vi "Cutoff Small Parts.vi"(8 "error in":errorcluster, 10 "Cutoff":dbl, 11 "Vec3d in":refnum<class "Vec3d.lvclass">) -> (0 "error out":errorcluster, 3 "Vec3d out":refnum<class "Vec3d.lvclass">)   [LabVIEW 2022 SP3, in "Vec3d.lvclass"]
uses:
  Vec3d.lvclass
  Vec3d.lvclass/Vec3d.ctl
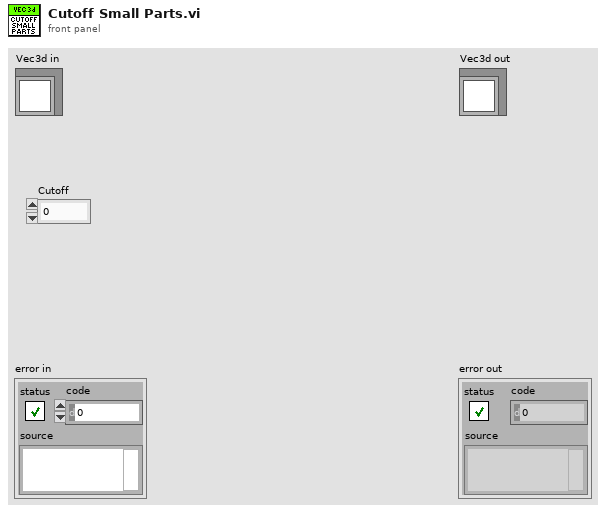
[diagram p1: front panel]
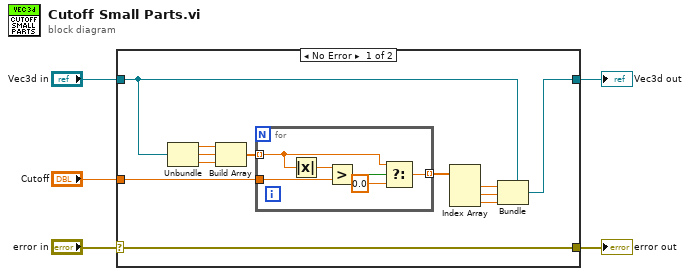
[diagram p0: block diagram]
diagram:
  n1 = case shown="No Error" "error in" {
    selector: "error in" -> [w17 w25]
    tunnel: [w17 w25] -> w4
    tunnel: [w9 w24] -> w2
    tunnel: "Vec3d in" -> [w10 w24]
    tunnel: "Cutoff" -> [w12 _]
    frame No Error {
      n2 = Unbundle(w10) -> (w16:dbl, w15:dbl, w14:dbl)
      n3 = Build Array(w16, w15, w14) -> (w13:dbl[])
      n4 = for {
        tunnel: w13 -> [w19] mode=indexing
        tunnel: w12 -> [w23]
        tunnel: [w20] -> w11 mode=indexing
        n5 = Absolute Value(x=w19) -> (abs(x)=w18:dbl)
        n6 = Greater?(x=w18, y=w23) -> (0:w22:bool)
        n7 = Select(t=w19, s=w22, f=0.0) -> (s? t:f=w20:dbl)
      }
      n8 = Index Array(array=w11) -> (element #1=w8:dbl, element #2=w7:dbl, element #3=w6:dbl)  [unwired: 3 in]
      n9 = Bundle(cluster=w10, w8, w7, w6) -> (w9:refnum<class "Vec3d.lvclass">)
    }
    frame Error {
    }
  }
  "error out" <- w4
  "Vec3d out" <- w2
